vi "Getinitiation.vi"(8 "error in (no error)":errorcluster, 11 "OneOfTemplate in":refnum<class "niswitch_grpc_ScanRequest_initiation_enum.lvclass">) -> (0 "error out":errorcluster, 2 "Get_Val":T1, 3 "OneOfTemplate out":refnum<class "niswitch_grpc_ScanRequest_initiation_enum.lvclass">)   [LabVIEW 2021, in "NI Switch_client.lvlib" / "niswitch_grpc_ScanRequest_initiation_enum.lvclass"]
uses:
  niswitch_grpc_ScanRequest_initiation_enum.lvclass
  niswitch_grpc_HandshakingInitiation.ctl
  niswitch_grpc_ScanRequest_initiation_enum.lvclass/niswitch_grpc_ScanRequest_initiation_enum.ctl
  NI Switch_client.lvlib
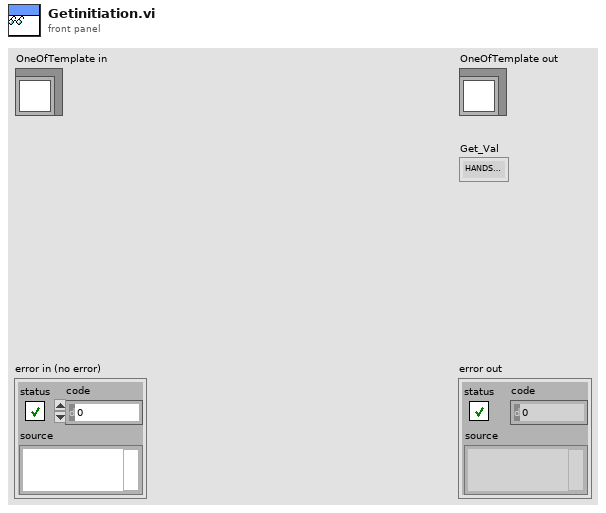
[diagram p1: front panel]
types:
  T1 = typedef "NI Switch_client.lvlib/niswitch_grpc_HandshakingInitiation.ctl" = enum32{"HANDSHAKING_INITIATION_NISWITCH_VAL_MEASUREMENT_DEVICE_INITIATED", "HANDSHAKING_INITIATION_NISWITCH_VAL_SWITCH_INITIATED"}
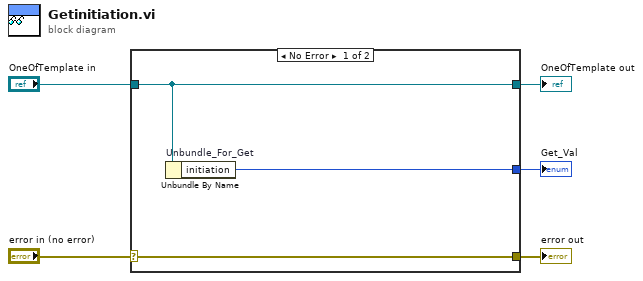
[diagram p0: block diagram]
diagram:
  n1 = case shown="No Error" "error in (no error)" {
    selector: "error in (no error)" -> [w8 w9]
    tunnel: [w8 w9] -> w4
    tunnel: [w7 w10] -> w2
    tunnel: "OneOfTemplate in" -> [w7 w10]
    tunnel: [w6 _] -> w1
    frame No Error {
      n2 = Unbundle By Name "Unbundle_For_Get"(w7) -> ("initiation"=w6:T1)
    }
    frame Error {
    }
  }
  "error out" <- w4
  "OneOfTemplate out" <- w2
  "Get_Val" <- w1
